vi "430_TCP_Close.vi"(2 "error in (no error)":errorcluster, 3 "connection ID":refnum<k5>) -> (0 "error out":errorcluster, 1 "connection ID out":refnum<k5>)   [LabVIEW 2019]
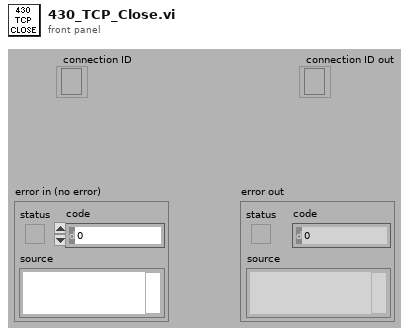
[diagram p1: front panel]
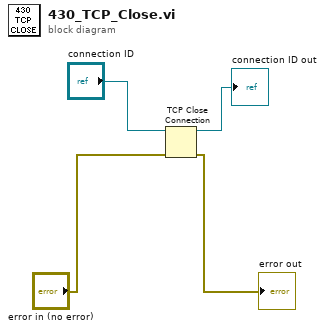
[diagram p0: block diagram]
diagram:
  n1 = TCP Close Connection(connection ID="connection ID", error in (no error)="error in (no error)") -> (connection ID out=→"connection ID out":refnum<k5>, error out=→"error out":errorcluster)  [unwired: 1 in]
